vi "Write Binary.vi"(6 "error in (no error)":errorcluster, 7 "Bytes":u8[](array[numeric]), 8 "timeout ms (5000)":i32=5000, 9 "RawSocket TCP Handler in":refnum<class "RawSocket TCP Handler.lvclass">) -> (0 "error out":errorcluster, 3 "RawSocket TCP Handler out":refnum<class "RawSocket TCP Handler.lvclass">)   [LabVIEW 2020, in "wamplv.lvlib" / "RawSocket TCP Handler.lvclass"]
uses:
  RawSocket TCP Handler.lvclass
  TypeDefs/Message Type.ctl
  RawSocket TCP Handler.lvclass/RawSocket TCP Handler.ctl
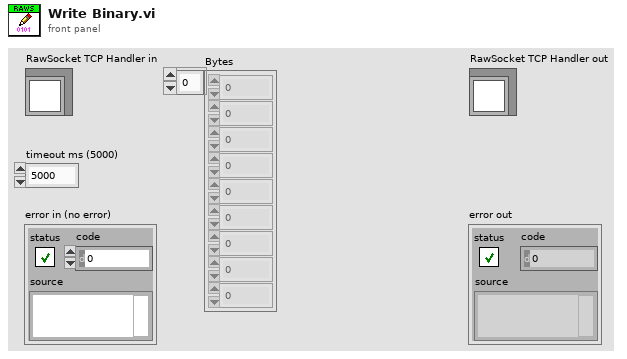
[diagram p1: front panel]
types:
  T1 = typedef "wamplv.lvlib/RawSocket TCP Handler.lvclass/Message Type.ctl" = enum8{"Regular WAMP message", "PING", "PONG"}
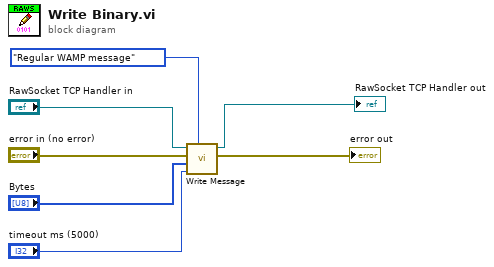
[diagram p0: block diagram]
diagram:
  n1 = call-dynamic "Write Message.vi"("Message Type"=Message_Type."Regular WAMP message", "timeout ms (5000)"="timeout ms (5000)", "Message"="Bytes", "error in (no error)"="error in (no error)", "RawSocket Handler in"="RawSocket TCP Handler in") -> ("error out"=→"error out":errorcluster, "RawSocket Handler out"=→"RawSocket TCP Handler out":refnum<class "RawSocket TCP Handler.lvclass">)  [unwired: 5 in]
